vi "HapticSPM_interactive_test-bench.vi"() -> ()   [LabVIEW 2022 SP3]
uses:
  <vilib>/Utility/sysdir.llb/System Directory Type.ctl
  Haptic-Programming-Interface/LabVIEW VIs/Haptic Prog Interface/Haptic Prog Interface.lvlib
panel:
  out "Waveform Graph":waveform(dbl)[](graph)
  out "Force Value":dbl[](graph)
  out "Signal Value (Scaled)":dbl[](graph)
  in  "Mode Selection":string(combo)="2" caption="Combo Box"
  in  "Suggested Settings":bool=TRUE
  in  "Cursor":bool=TRUE
  out "?":bool=TRUE
  out "data":dbl[][](array[numeric])
  in  "Tab Control":enum32{"2 atoms", "1 atom", "Line", "N"}(tab)
  out "Frame Properties (m)":T1
  in  "Function":string(combo)="0" caption="Combo Box"
  in  "Gain (mm/pm)":dbl=2.0 caption="Numeric" format="%.1g"
  in  "k":dbl=0.6000000000000001 caption="Numeric" step=0.1 format="%.1g"
  in  "Setpoint":dbl=8.000000413701856e-11 caption="Numeric" step=1e-11 format="%.0p"
  in  "Gain":dbl=1.0 caption="Numeric" format="%.1g"
  out "Value":dbl caption="Numeric" format="%#_2p"
  out "Surf Loc (m)":dbl
  out "Forces":T2 {"Fz (N)" format="%.1f"; "Fy (N)" format="%.1f"; "Fx (N)" format="%.1f"}
  out "Position (Reframed)":cluster{"x (m)":dbl, "y (m)":dbl, "z (mm)":dbl} {"z (mm)" format="%.0p"; "y (m)" format="%.1p"; "x (m)" format="%.1p"}
  # "Super Ultra Mega Haptic SPM Controller 3000"
  # "Signal"
  # "Force"
  # "Surface Scale"
  # "Move pen in all three dimensions to calibrate"
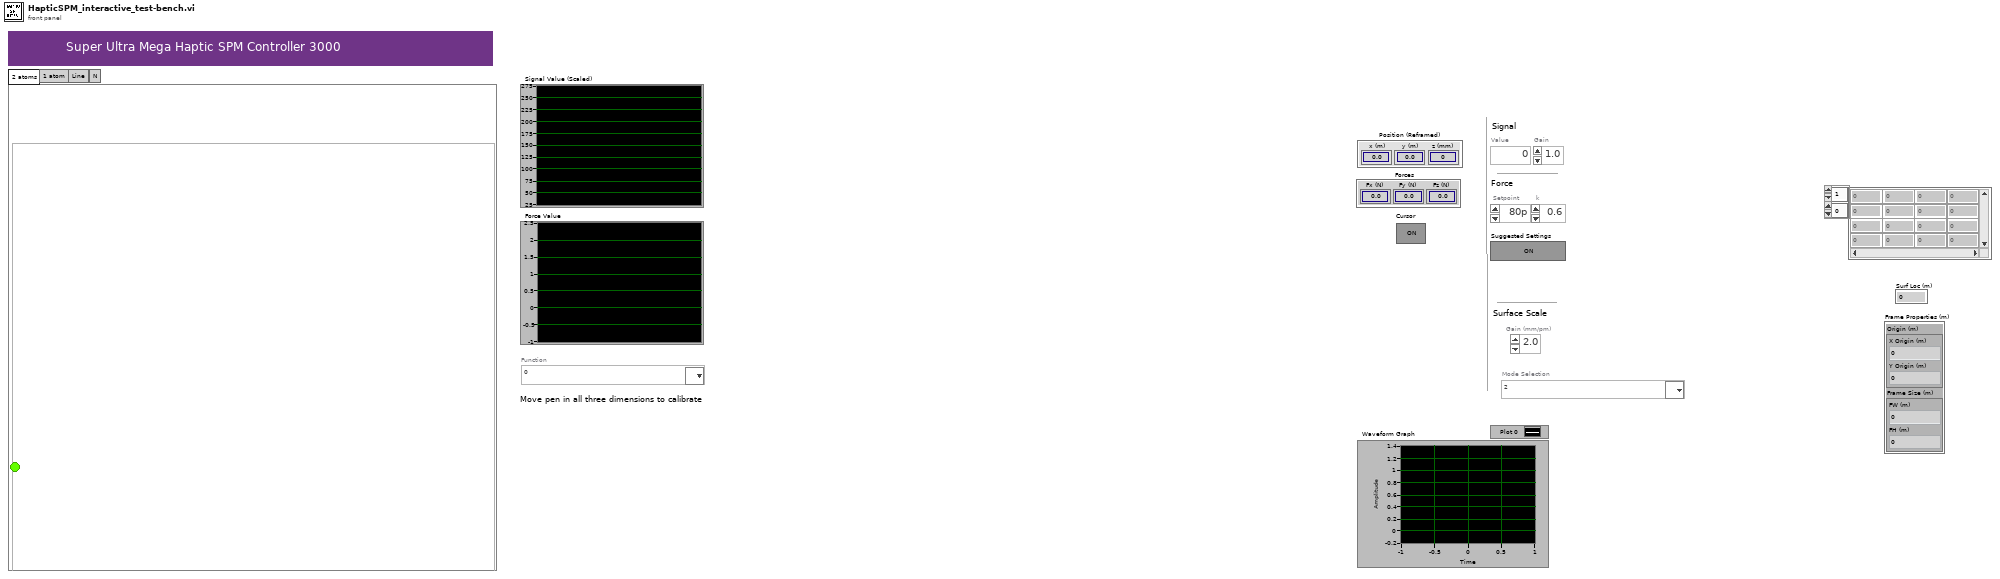
[diagram p1: front panel]
types:
  T1 = cluster{"Origin (m)":cluster{"X Origin (m)":dbl, "Y Origin (m)":dbl}, "Frame Size (m)":cluster{"FW (m)":dbl, "FH (m)":dbl}}
  T2 = cluster{"Fx (N)":dbl, "Fy (N)":dbl, "Fz (N)":dbl}
  T3 = cluster{"kx (N/m)":dbl, "ky (N/m)":dbl, "kz (N/m)":dbl}
  T4 = cluster{"X Drag":bool, "Y Drag":bool, "Z Drag":bool}
  T5 = cluster{"x (mm)":dbl, "y (mm)":dbl, "z (mm)":dbl}
  T6 = typedef "System Directory Type.ctl" = i32
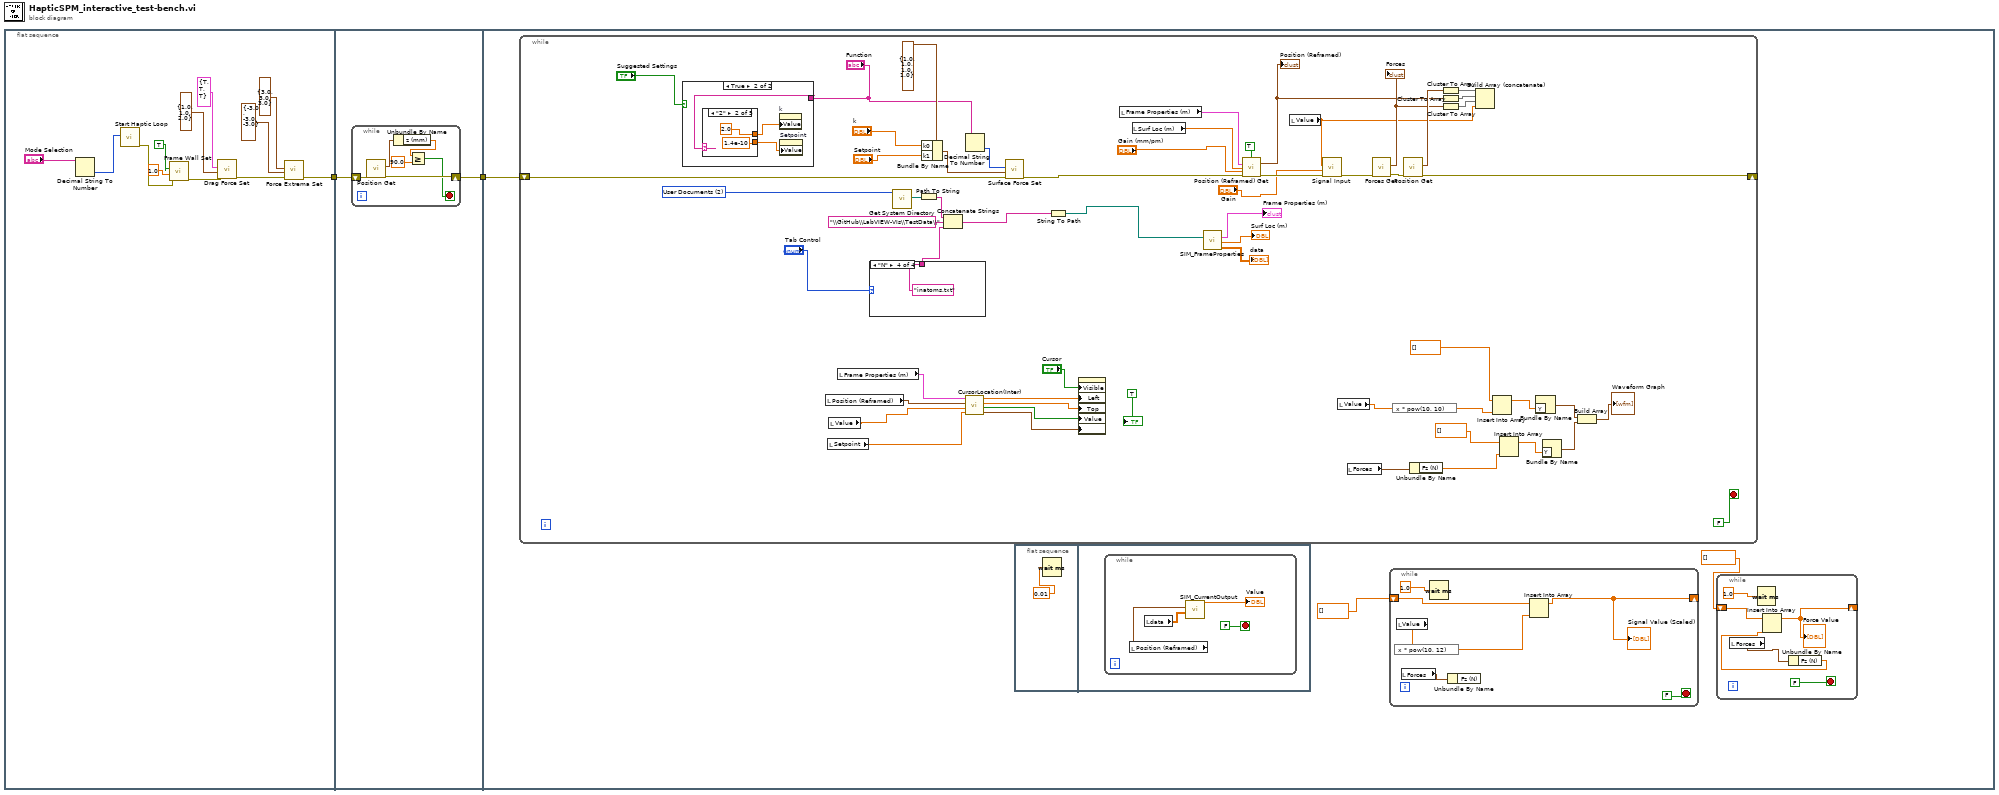
[diagram p0: block diagram]
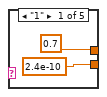
[diagram p3: hidden frame]
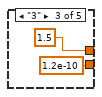
[diagram p4: hidden frame]
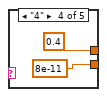
[diagram p5: hidden frame]
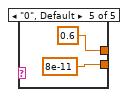
[diagram p6: hidden frame]
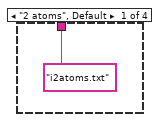
[diagram p7: hidden frame]
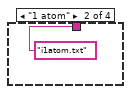
[diagram p8: hidden frame]
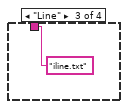
[diagram p9: hidden frame]
diagram:
  n1 = flat-sequence {
    tunnel: [w13] -> w2
    tunnel: w2 -> [w16]
    tunnel: [w15] -> w1
    tunnel: w1 -> [w25]
    frame #0 {
      n2 = Decimal String To Number(string="Mode Selection") -> (number=w3:i32)  [unwired: 2 in, 1 out]
      n3 = call "Start Haptic Loop.vi"("Mode Selection"=w3) -> ("error out"=w5:errorcluster)  [unwired: 10 in]
      n4 = call "Frame Wall Set.vi"("error in (no error)"=w5, "Wall Stiffness (N/m)"=1.0 ("Wall Stiffness"), "Restrict to Frame"=TRUE) -> ("error out"=w6:errorcluster)  [unwired: 8 in]
      n5 = call "Drag Force Set.vi"("error in (no error)"=w6, "Drag Coefficients (N/m)"=T3 {"kx (N/m)"=1.0, "ky (N/m)"=1.0, "kz (N/m)"=2.0} ("Drag Coefficients"), "Drag Force Toggles"=T4 {"X Drag"=TRUE, "Y Drag"=TRUE, "Z Drag"=TRUE}) -> ("error out"=w14:errorcluster)  [unwired: 8 in]
      n6 = call "Force Extrema Set.vi"("error in (no error)"=w14, "Minimum Force (N)"=T2 {"Fx (N)"=-3.0, "Fy (N)"=-3.0, "Fz (N)"=-3.0} ("Minimum Force"), "Maximum Force (N)"=T2 {"Fx (N)"=3.0, "Fy (N)"=3.0, "Fz (N)"=3.0} ("Maximum Force")) -> ("error out"=w13:errorcluster)  [unwired: 8 in]
    }
    frame #1 {
      n7 = while {
        shift-right: [w21] -> w15
        shift-left: w16 -> [w22]
        stop <- w17 stop-if-true
        n8 = call "Position Get.vi"("error in (no error)"=w22) -> ("error out"=w21:errorcluster, "Position"=w20:T5)  [unwired: 9 in]
        n9 = Unbundle By Name(w20) -> ("z (mm)"=w19:dbl)
        n10 = Greater Or Equal?(x=w19, y=90.0) -> (x >= y?=w17:bool)
      }
    }
    frame #2 {
      n11 = while {
        shift-right: [w55] -> _
        shift-left: w25 -> [w101]
        stop <- FALSE stop-if-true
        w80 = T6 2 items=["User Home"=0, "User Desktop"=1, "User Documents"=2, "User Application Data"=3, "User Preferences"=4, "User Temporary"=5, "Public Documents"=6, "Public Application Data"=7, "Public Preferences"=8, "Public Cache"=13, "System Core Libraries"=9, "System Installed Libraries"=10, "Application Files"=11, "Boot Volume Root"=12] ("system directory type")
        n12 = case shown="True" "Suggested Settings" {
          tunnel: "Function" -> [_ w102]
          frame False {
          }
          frame True {
            n13 = case shown="\"2\"" w102 {
              tunnel: [0.7 2.0 1.5 0.4 0.6] -> w104
              tunnel: [2.4e-10 1.4e-10 1.2e-10 8e-11 8e-11] -> w103
              frame "1" {
              }
              frame "2" {
              }
              frame "3" {
              }
              frame "4" {
              }
              frame "0", Default {
              }
            }
            n14 = property on="k" class="DigNum (strict)"("Value"=w104) -> ()  [unwired: 2 in, 2 out]
            n15 = property on="Setpoint" class="DigNum (strict)"("Value"=w103) -> ()  [unwired: 2 in, 2 out]
          }
        }
        n16 = local read "Position (Reframed)"() -> (w70:cluster{"x (m)":dbl, "y (m)":dbl, "z (mm)":dbl})
        n17 = local read "Setpoint"() -> (w68:dbl)
        n18 = local read "Value"() -> (w69:dbl)
        n19 = local read "Frame Properties (m)"() -> (w71:T1)
        n20 = case shown="\"N\"" "Tab Control" {
          tunnel: ["i2atoms.txt" "i1atom.txt" "iline.txt" "inatoms.txt"] -> w61
          frame "2 atoms", Default {
          }
          frame "1 atom" {
          }
          frame "Line" {
          }
          frame "N" {
          }
        }
        n21 = call <vilib>:"Get System Directory.vi"("system directory type"=w80) -> ("system directory"=w79:path)  [unwired: 10 in]
        n22 = Path To String(path=w79) -> (string=w78:string)
        n23 = Bundle By Name(cluster=cluster{"k0":dbl, "k1":dbl, "k2":dbl, "k3":dbl} {"k0"=1.0, "k1"=1.0, "k2"=1.0, "k3"=1.0} ("Force Constants"), "k0"="k", "k1"="Setpoint") -> (w94:cluster{"k0":dbl, "k1":dbl, "k2":dbl, "k3":dbl})
        n24 = Concatenate Strings(w78, "\\GitHub\\LabVIEW-VIs\\TestData\\" ("string"), w61) -> (w76:string)
        n25 = call "CursorLocation(Inter).vi"("Setpoint"=w68, "Value"=w69, "Position (Reframed)"=w70, "Frame Properties (m)"=w71) -> ("Cursor Size"=w64:cluster{"Width":i32, "Height":i32}, "Current Above Setpoint?"=w65:bool, "Y-Coordinate"=w66:dbl, "X-Coordinate"=w67:dbl)
        n26 = Decimal String To Number(string="Function") -> (number=w93:i32)  [unwired: 2 in, 1 out]
        n27 = call "Surface Force Set.vi"("error in (no error)"=w101, "Force Constants"=w94, "Force Settings"=w93) -> ("error out"=w82:errorcluster)  [unwired: 8 in]
        n28 = String To Path(string=w76) -> (path=w74:path)
        n29 = property class="Bool (strict)"("Visible"="Cursor", "Left"=w67, "Top"=w66, "Value"=w65, "Button Size"=w64) -> ()  [unwired: 2 in, 2 out]
        n30 = local read "Frame Properties (m)"() -> (w83:T1)
        n31 = local read "Surf Loc (m)"() -> (w99:dbl)
        n32 = call "SIM_FrameProperties.vi"("file path (dialog if empty)"=w74) -> ("data"=→"data":dbl[][], "Surf Loc (m)"=→"Surf Loc (m)":dbl, "Frame Properties (m)"=→"Frame Properties (m)":T1)  [unwired: 8 in]
        n33 = call "Position (Reframed) Get.vi"("Z Rescaling"=TRUE, "Frame Properties (m)"=w83, "Surface Location (m)"=w99, "Scaling (mm per pm)"="Gain (mm/pm)", "error in (no error)"=w82) -> ("Reframed Position (m)"=w73:cluster{"x (m)":dbl, "y (m)":dbl, "z (m)":dbl}, "error out"=w97:errorcluster)  [unwired: 9 in]
        "Position (Reframed)" <- w73
        n34 = local read "Value"() -> (w86:dbl)
        n35 = call "Signal Input.vi"("error in (no error)"=w97, "Gain"="Gain", "Signal"=w86) -> ("error out"=w98:errorcluster)  [unwired: 8 in]
        n36 = local read "Value"() -> (w54:dbl)
        n37 = local read "Forces"() -> (w53:T2)
        n38 = call "Forces Get.vi"("error in (no error)"=w98) -> ("error out"=w96:errorcluster, "Force (N)"=w88:T2)  [unwired: 9 in]
        "Forces" <- w88
        n39 = expression code="x * pow(10, 10)"(w54) -> (w51:dbl)
        n40 = call "Position Get.vi"("error in (no error)"=w96) -> ("error out"=w55:errorcluster, "Position"=w91:T5)  [unwired: 9 in]
        n41 = Unbundle By Name(w53) -> ("Fz (N)"=w48:dbl)
        n42 = Cluster To Array(cluster=w91) -> (array=w90:dbl[])
        n43 = Cluster To Array(cluster=w73) -> (array=w89:dbl[])
        n44 = Cluster To Array(cluster=w88) -> (array=w87:dbl[])
        n45 = Build Array (concatenate)(w90, w89, w87, w86) -> ()  [unwired: 1 out]
        n46 = Insert Into Array(array=dbl[] [], new element=w51) -> (w50:dbl[])  [unwired: 1 in]
        n47 = Insert Into Array(array=dbl[] [], new element=w48) -> (w47:dbl[])  [unwired: 1 in]
        n48 = Bundle By Name("Y"=w50) -> (w46:waveform(dbl))  [unwired: 1 in]
        n49 = Bundle By Name("Y"=w47) -> (w45:waveform(dbl))  [unwired: 1 in]
        n50 = Build Array(w46, w45) -> (→"Waveform Graph":waveform(dbl)[])
        "?" <- TRUE
      }
      n51 = flat-sequence {
        frame #0 {
          n52 = Wait (ms)(milliseconds to wait=0.01) -> ()  [unwired: 1 out]
        }
        frame #1 {
          n53 = while {
            stop <- FALSE stop-if-true
            n54 = local read "Position (Reframed)"() -> (w40:cluster{"x (m)":dbl, "y (m)":dbl, "z (mm)":dbl})
            n55 = local read "data"() -> (w41:dbl[][])
            n56 = call "SIM_CurrentOutput.vi"("array"=w41, "Position (Reframed)"=w40) -> ("Current Out (A)"=→"Value":dbl)  [unwired: 8 in, 1 out]
          }
        }
      }
      n57 = while {
        shift-right: [w32] -> _
        shift-left: dbl[] [] ("element") -> [w34]
        stop <- FALSE stop-if-true
        n58 = local read "Value"() -> (w38:dbl)
        n59 = expression code="x * pow(10, 12)"(w38) -> (w33:dbl)
        n60 = local read "Forces"() -> (w35:T2)
        n61 = Wait (ms)(milliseconds to wait=1.0) -> ()  [unwired: 1 out]
        n62 = Unbundle By Name(w35) -> ()  [unwired: 1 out]
        n63 = Insert Into Array(array=w34, new element=w33) -> (w32:dbl[])  [unwired: 1 in]
        "Signal Value (Scaled)" <- w32
      }
      n64 = while {
        shift-right: [w31] -> _
        shift-left: dbl[] [] ("element") -> [w30]
        stop <- FALSE stop-if-true
        n65 = local read "Forces"() -> (w26:T2)
        n66 = Wait (ms)(milliseconds to wait=1.0) -> ()  [unwired: 1 out]
        n67 = Unbundle By Name(w26) -> ("Fz (N)"=w27:dbl)
        n68 = Insert Into Array(array=w30, new element=w27) -> (w31:dbl[])  [unwired: 1 in]
        "Force Value" <- w31
      }
    }
  }
